vi "Set Home Preset Position.vi"(4 "error in (no error)":errorcluster, 5 "Home Preset Position (0 units)":dbl format="%.4g", 6 "Axis (1)":i32=1 min=1 max=3, 7 "VISA resource name":refnum<visa-resource-name>) -> (0 "error out":errorcluster, 3 "VISA resource name out":refnum<visa-resource-name>)   [LabVIEW 2019, in "Newport ESP301.lvlib"]
doc: "This command defines the value that is loaded in the position counter when home is found. The default value for all motion devices is 0. This means that unless a new value is defined using this command, the home position will be set to 0 when a home search is initiated using the OR command or from the front panel (if available).\nNote:\nThe change takes effect only when a subsequent home search routine is performed. To make the change permanent, use the \"Save Settings To Non-Volatile Memory.vi\"."
uses:
  Newport ESP301.lvlib
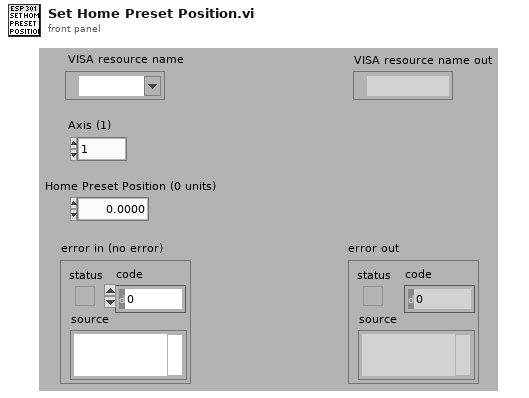
[diagram p1: front panel]
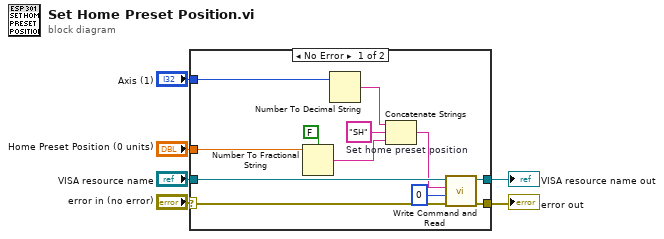
[diagram p0: block diagram]
diagram:
  n1 = case shown="No Error" "error in (no error)" {
    selector: "error in (no error)" -> [w9 w20]
    tunnel: [w7 w20] -> w6
    tunnel: "VISA resource name" -> [w12 w19]
    tunnel: [w8 w19] -> w5
    tunnel: "Axis (1)" -> [w16 _]
    tunnel: "Home Preset Position (0 units)" -> [w15 _]
    frame No Error {
      w18 = "SH"  # Set home preset position
      n2 = Number To Fractional String(use system decimal point (T)=FALSE ("utiliser le séparateur décimal du système (V)"), number=w15) -> (F-format string=w14:string)  [unwired: 2 out]
      n3 = Number To Decimal String(number=w16) -> (decimal integer string=w17:string)  [unwired: 1 out]
      n4 = Concatenate Strings(w17, w18, w14) -> (w11:string)
      n5 = call "Write Command and Read.vi"("error in (no error)"=w9, "Bytes to read (100)"=u32 0, "Command"=w11, "VISA resource name"=w12) -> ("error out"=w7:errorcluster, "VISA resource name out"=w8:refnum<visa-resource-name>)  [unwired: 1 in, 3 out]
    }
    frame Error {
    }
  }
  "error out" <- w6
  "VISA resource name out" <- w5
